vi "Perdite da step carichi.vi"(5 "k0":dbl=1.0 format="%#_13g", 7 "Scorr 0":dbl, 8 "Acqisizioni termica":T4, 9 "Perdite da termica":T6, 10 "Acquisizioni step carichi":T5, 11 "Perdite da prova a vuoto 2":T1) -> (1 "RISULTATI":T2, 2 "Calcoli da step carichi":T3)   [LabVIEW 2019]
uses:
  <vilib>/Analysis/NI_AALPro.lvlib
panel:
  out "Array 4":dbl[](array[numeric])
  out "Array 3":dbl[](array[numeric])
  out "R iniz carico":dbl
  out "slope":dbl
  out "intercept":dbl
  out "XY Graph":cluster{dbl[], "Best Linear Fit":dbl[]}[](graph)
  out "Array 2":dbl[](array[numeric])
  out "Array":dbl[](array[numeric])
  out "size(s) 2":i32
  out "size(s)":i32
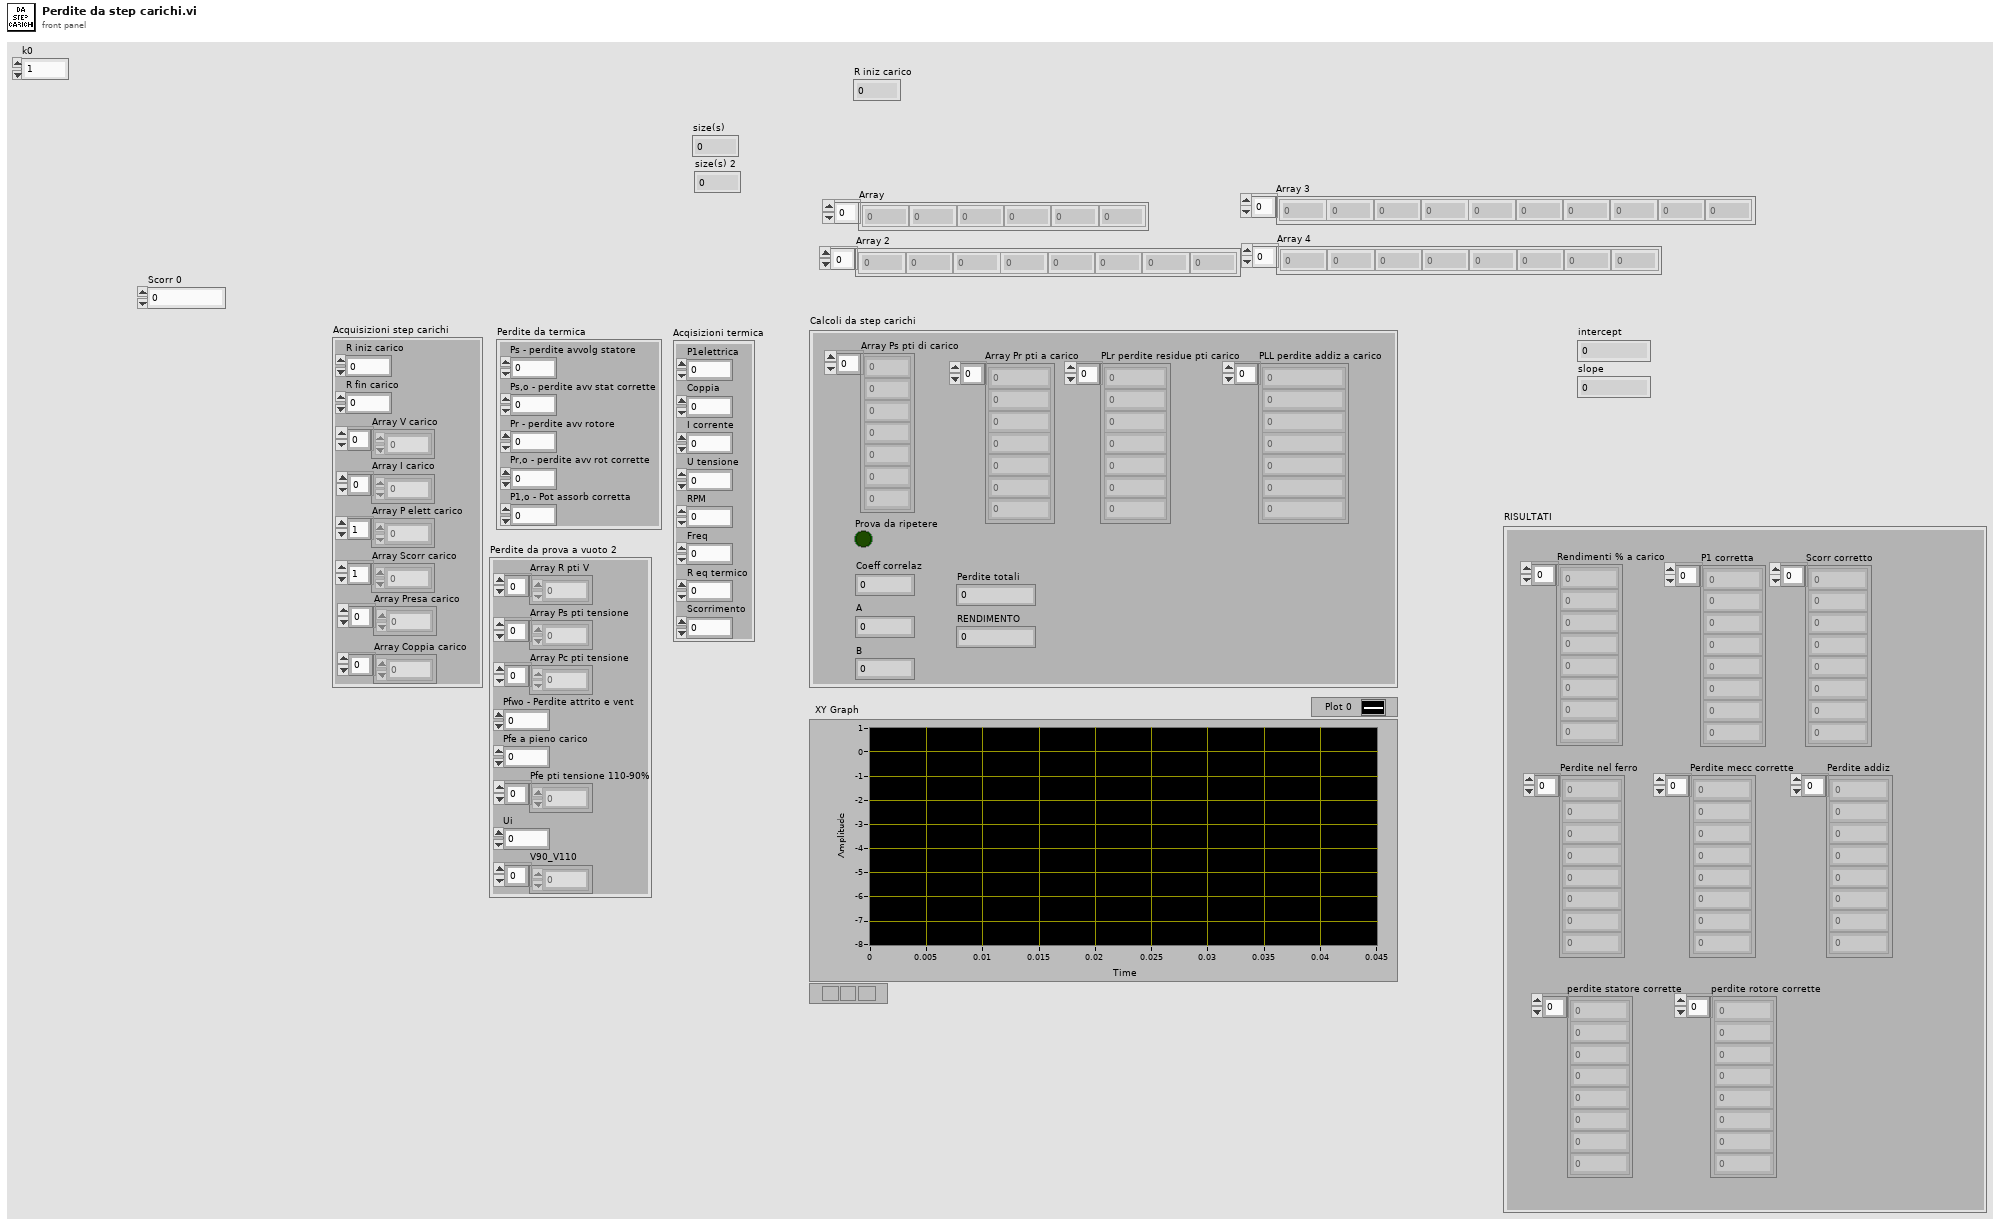
[diagram p1: front panel]
types:
  T1 = cluster{"Array R pti V":dbl[], "Array Ps pti tensione":dbl[], "Array Pc pti tensione":dbl[], "Pfwo - Perdite attrito e vent":dbl, "Pfe a pieno carico":dbl, "Pfe pti tensione 110-90% ":dbl[], "Ui":dbl, "V90_V110":dbl[]}
  T2 = cluster{"Rendimenti % a carico":dbl[], "P1 corretta":dbl[], "Scorr corretto":dbl[], "Perdite nel ferro":dbl[], "Perdite mecc corrette":dbl[], "Perdite addiz":dbl[], "perdite statore corrette":dbl[], "perdite rotore corrette":dbl[]}
  T3 = cluster{"Array Ps pti di carico":dbl[], "Array Pr pti a carico":dbl[], "PLr perdite residue pti carico":dbl[], "A":dbl, "B":dbl, "Coeff correlaz":dbl, "Prova da ripetere":bool, "PLL perdite addiz a carico":dbl[], "Perdite totali":dbl, "RENDIMENTO":dbl}
  T4 = cluster{"P1elettrica":dbl, "Coppia":dbl, "I corrente":dbl, "U tensione":dbl, "RPM":dbl, "Freq":dbl, "R eq termico":dbl, "Scorrimento":dbl}
  T5 = cluster{"R iniz carico":dbl, "R fin carico":dbl, "Array V carico":dbl[], "Array I carico":dbl[], "Array P elett carico":dbl[], "Array Scorr carico":dbl[], "Array Presa carico":dbl[], "Array Coppia carico":dbl[]}
  T6 = cluster{"Ps - perdite avvolg statore":dbl, "Ps,o - perdite avv stat corrette":dbl, "Pr - perdite avv rotore":dbl, "Pr,o - perdite avv rot corrette":dbl, "P1,o - Pot assorb corretta":dbl}
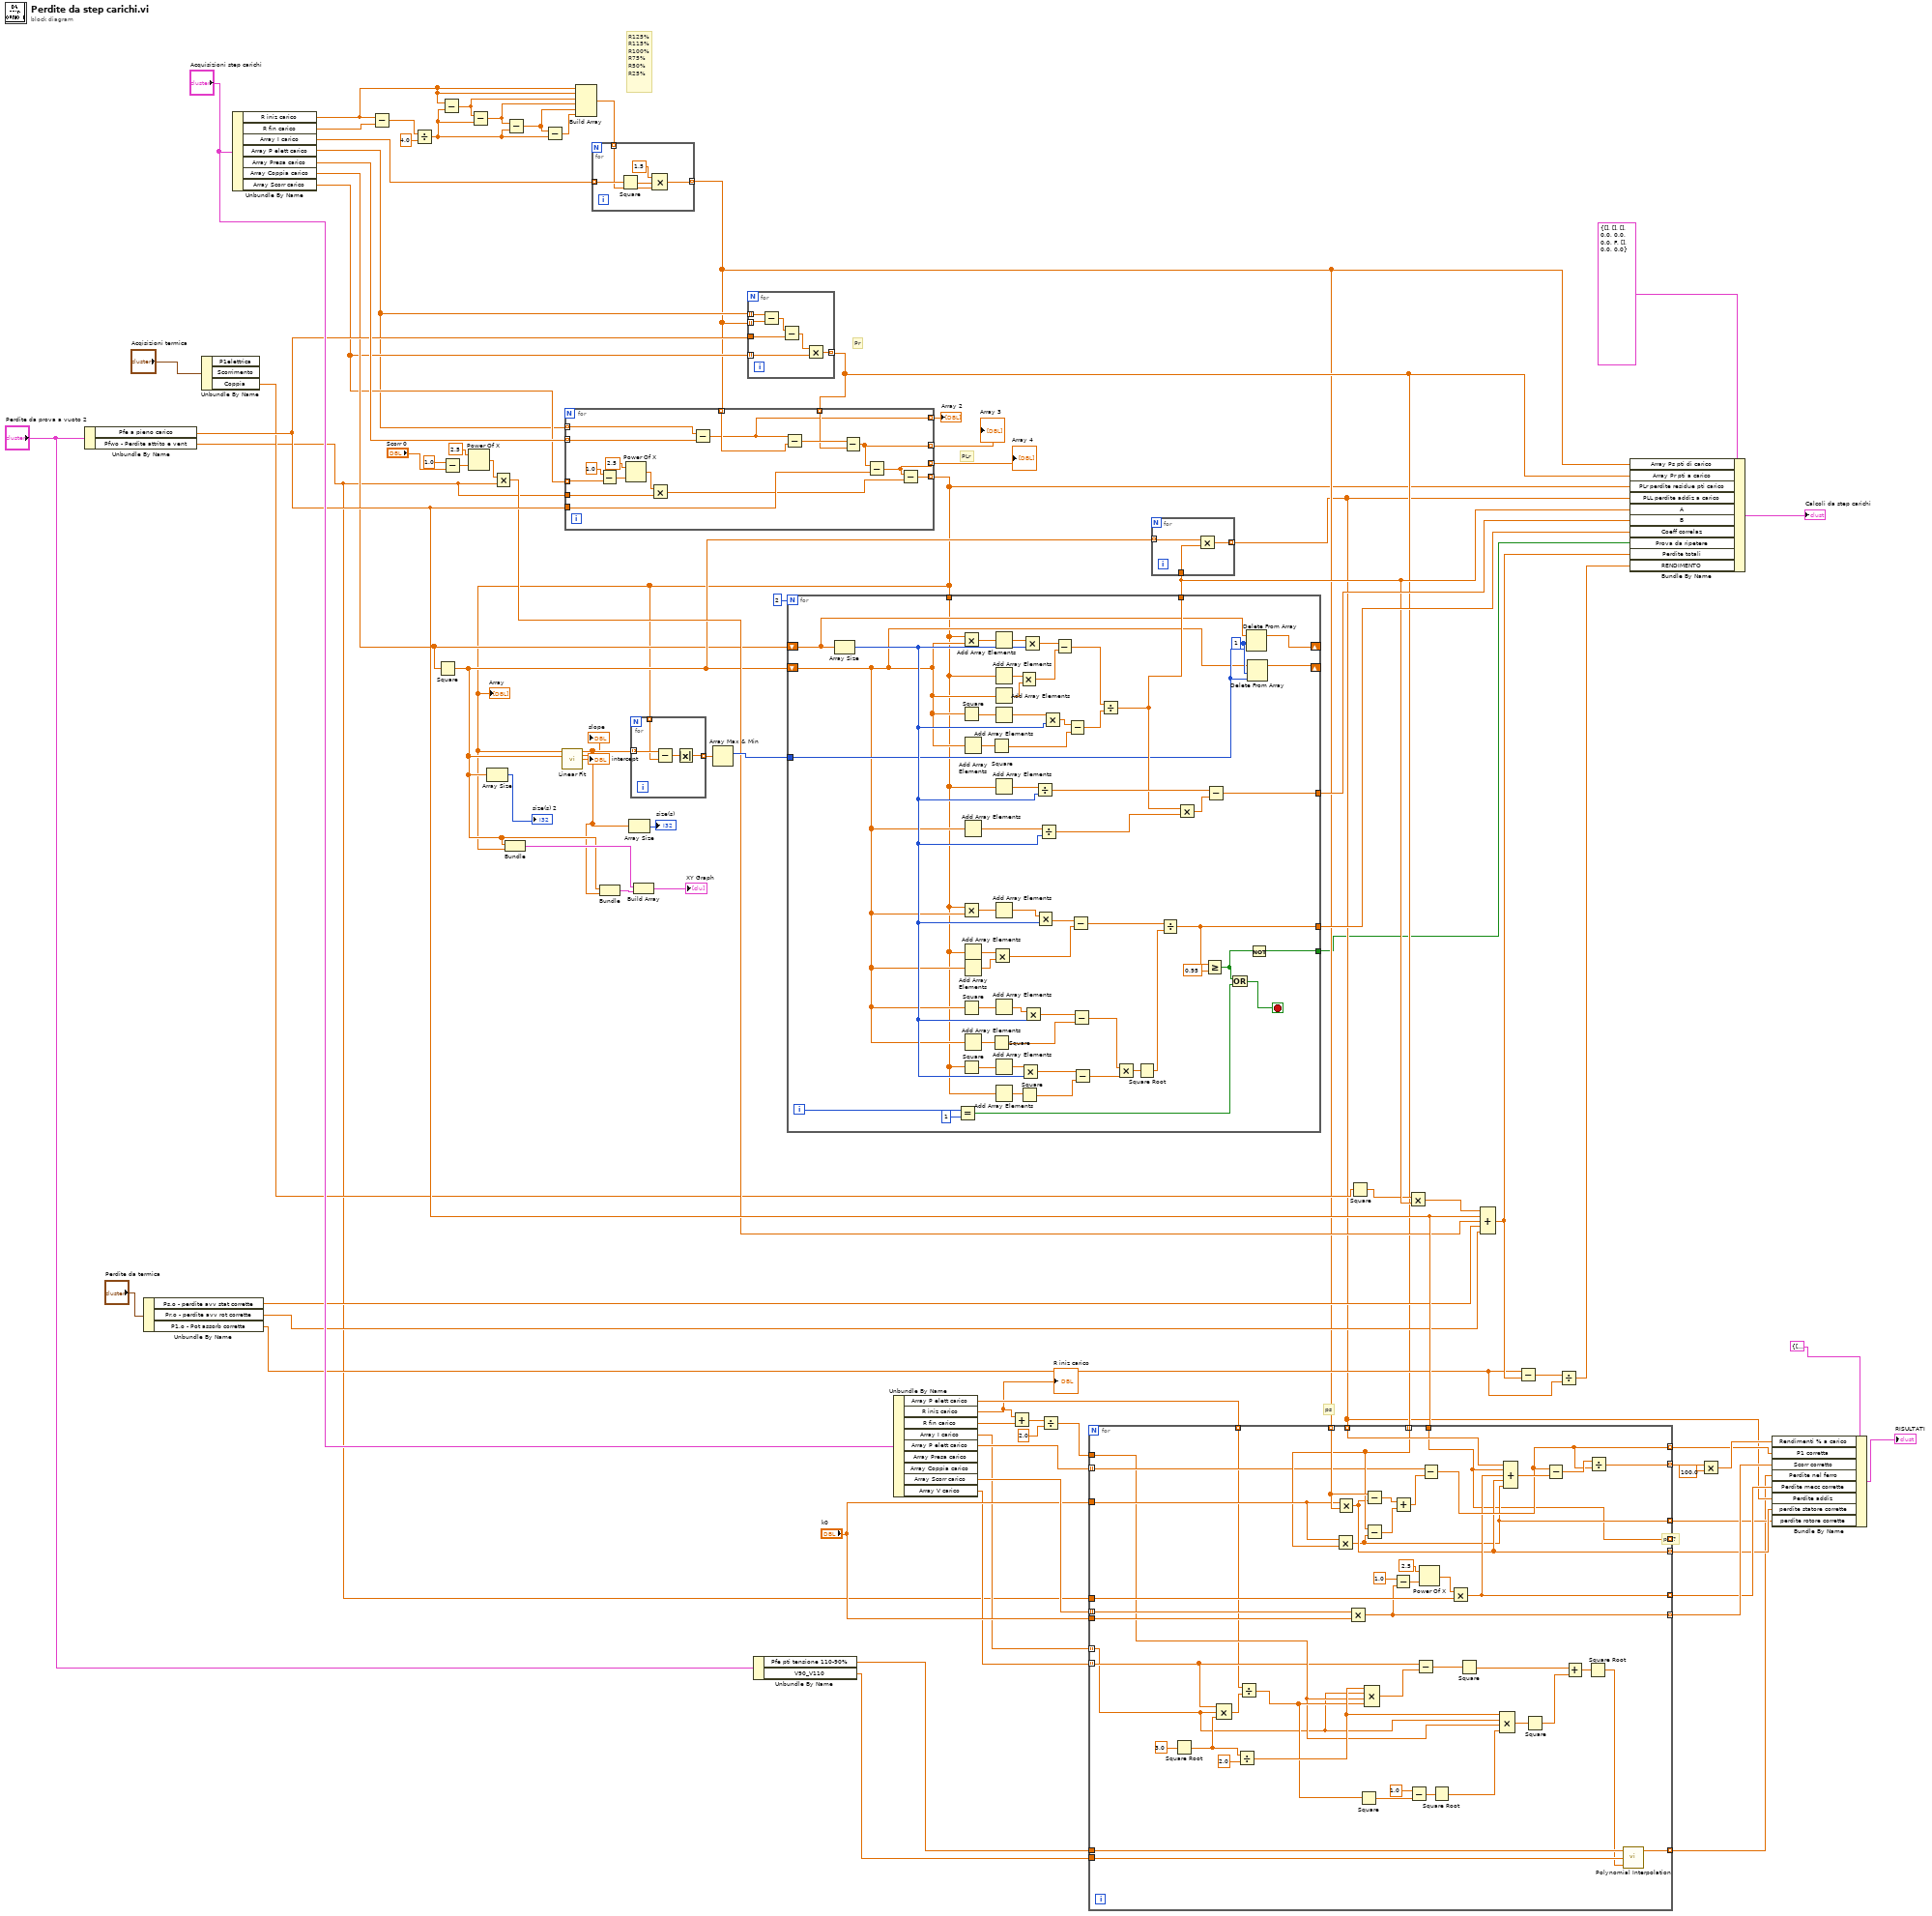
[diagram p0: block diagram]
diagram:
  # "pfe?"
  # "ps"
  # "PLr"
  # "Pr"
  # "R125%\nR115%\nR100%\nR75%\nR50%\nR25%"
  n1 = Unbundle By Name("Perdite da prova a vuoto 2") -> ("Pfe a pieno carico"=w47:dbl, "Pfwo - Perdite attrito e vent"=w1:dbl)
  n2 = Unbundle By Name("Perdite da termica") -> ("Ps,o - perdite avv stat corrette"=w43:dbl, "Pr,o - perdite avv rot corrette"=w42:dbl, "P1,o - Pot assorb corretta"=w41:dbl)
  n3 = Unbundle By Name("Acqisizioni termica") -> ("Coppia"=w45:dbl)  [unwired: 2 out]
  n4 = Unbundle By Name("Acquisizioni step carichi") -> ("R iniz carico"=w70:dbl, "R fin carico"=w69:dbl, "Array I carico"=w68:dbl[], "Array P elett carico"=w34:dbl[], "Array Presa carico"=w65:dbl[], "Array Coppia carico"=w36:dbl[], "Array Scorr carico"=w35:dbl[])
  n5 = Subtract(x=w70, y=w69) -> (x-y=w85:dbl)
  n6 = Divide(x=w85, y=4.0) -> (x/y=w57:dbl)
  n7 = Square(x=w36) -> (x^2=w40:dbl[])
  n8 = Subtract(x=w70, y=w57) -> (x-y=w83:dbl)
  n9 = Subtract(x=1.0, y="Scorr 0") -> (x-y=w79:dbl)
  n10 = Power Of X(1:w79, 2:2.5 ("y")) -> (0:w77:dbl)
  n11 = Subtract(x=w83, y=w57) -> (x-y=w82:dbl)
  n12 = Array Size(array=w40) -> (size(s)=→"size(s) 2":i32)
  n13 = Multiply(x=w77, y=w1) -> (x*y=w46:dbl)
  n14 = Subtract(x=w82, y=w57) -> (x-y=w58:dbl)
  n15 = Subtract(x=w58, y=w57) -> (x-y=w56:dbl)
  n16 = Build Array(w70, w70, w83, w82, w58, w56) -> (w81:dbl[])
  n17 = for {
    tunnel: w68 -> [w89] mode=indexing
    tunnel: w81 -> [w88] mode=indexing
    tunnel: [w87] -> w29 mode=indexing
    n18 = Square(x=w89) -> (x^2=w86:dbl)
    n19 = Compound Arithmetic op=MULTIPLY(1.5 ("value"), w86, w88) -> (w87:dbl)
  }
  n20 = for {
    tunnel: w34 -> [w97] mode=indexing
    tunnel: w29 -> [w96] mode=indexing
    tunnel: w47 -> [w94]
    tunnel: [w91] -> w31 mode=indexing
    tunnel: w35 -> [w92] mode=indexing
    n21 = Subtract(x=w97, y=w96) -> (x-y=w95:dbl)
    n22 = Subtract(x=w95, y=w94) -> (x-y=w93:dbl)
    n23 = Multiply(x=w93, y=w92) -> (x*y=w91:dbl)
  }
  n24 = for {
    tunnel: w34 -> [w114] mode=indexing
    tunnel: w65 -> [w113] mode=indexing
    tunnel: w29 -> [w112] mode=indexing
    tunnel: w31 -> [w110] mode=indexing
    tunnel: w47 -> [w108]
    tunnel: [w109] -> w17 mode=indexing
    tunnel: w35 -> [w103] mode=indexing
    tunnel: w1 -> [w102]
    tunnel: [w100] -> w54 mode=indexing
    tunnel: [w99] -> w3 mode=indexing
    tunnel: [w98] -> w2 mode=indexing
    n25 = Subtract(x=1.0, y=w103) -> (x-y=w105:dbl)
    n26 = Power Of X(1:w105, 2:2.5 ("y")) -> (0:w107:dbl)
    n27 = Multiply(x=w107, y=w102) -> (x*y=w101:dbl)
    n28 = Subtract(x=w114, y=w113) -> (x-y=w100:dbl)
    n29 = Subtract(x=w100, y=w112) -> (x-y=w111:dbl)
    n30 = Subtract(x=w111, y=w110) -> (x-y=w99:dbl)
    n31 = Subtract(x=w99, y=w108) -> (x-y=w98:dbl)
    n32 = Subtract(x=w98, y=w101) -> (x-y=w109:dbl)
  }
  "Array" <- w17
  "Array 2" <- w54
  "Array 3" <- w3
  "Array 4" <- w2
  n33 = Bundle(w40, w17) -> (w53:cluster{dbl[], dbl[]})  [unwired: 1 in]
  n34 = call <vilib>:"Linear Fit.vi"("Y"=w17, "X"=w40) -> ("Best Linear Fit"=w39:dbl[], "slope"=→"slope":dbl, "intercept"=→"intercept":dbl)  [unwired: 9 in, 2 out]
  n35 = Bundle(w40, "Best Linear Fit"=w39) -> (w52:cluster{dbl[], "Best Linear Fit":dbl[]})  [unwired: 1 in]
  n36 = Array Size(array=w39) -> (size(s)=→"size(s)":i32)
  n37 = for {
    tunnel: w39 -> [w118] mode=indexing
    tunnel: w17 -> [w117] mode=indexing
    tunnel: [w115] -> w75 mode=indexing
    n38 = Subtract(x=w118, y=w117) -> (x-y=w116:dbl)
    n39 = Absolute Value(x=w116) -> (abs(x)=w115:dbl)
  }
  n40 = Build Array(w53, w52) -> (→"XY Graph":cluster{dbl[], "Best Linear Fit":dbl[]}[])
  n41 = Array Max & Min(array=w75) -> (max index (indices)=w74:i32)  [unwired: 3 out]
  n42 = Unbundle By Name("Perdite da prova a vuoto 2") -> ("Pfe pti tensione 110-90%"=w12:dbl[], "V90_V110"=w11:dbl[])
  n43 = for {
    N: 2 -> [_]
    tunnel: [w143] -> w48
    tunnel: w17 -> [w123]
    tunnel: [w119] -> w4
    tunnel: [w142] -> w63
    shift-right: [w138] -> _
    shift-left: w36 -> [w139]
    shift-right: [w137] -> _
    shift-left: w40 -> [w131]
    tunnel: w74 -> [w140]
    tunnel: [w128] -> w62
    i -> [w135]
    stop <- w132 stop-if-true
    w141 = 1 ("length")
    n44 = Array Size(array=w139) -> (size(s)=w146:i32)
    n45 = Equal?(x=w135, y=1) -> (x = y?=w133:bool)
    n46 = Square(x=w131) -> (x^2=w130:dbl[])
    n47 = Square(x=w131) -> (x^2=w153:dbl[])
    n48 = Square(x=w123) -> (x^2=w147:dbl[])
    n49 = Multiply(x=w123, y=w131) -> (x*y=w175:dbl[])
    n50 = Multiply(x=w123, y=w131) -> (x*y=w158:dbl[])
    n51 = Add Array Elements(numeric array=w131) -> (sum=w167:dbl)
    n52 = Add Array Elements(numeric array=w131) -> (sum=w162:dbl)
    n53 = Add Array Elements(numeric array=w123) -> (sum=w156:dbl)
    n54 = Add Array Elements(numeric array=w131) -> (sum=w155:dbl)
    n55 = Add Array Elements(numeric array=w131) -> (sum=w150:dbl)
    n56 = Square(x=w167) -> (x^2=w166:dbl)
    n57 = Square(x=w150) -> (x^2=w149:dbl)
    n58 = Multiply(x=w156, y=w155) -> (x*y=w154:dbl)
    n59 = Add Array Elements(numeric array=w175) -> (sum=w174:dbl)
    n60 = Add Array Elements(numeric array=w123) -> (sum=w172:dbl)
    n61 = Add Array Elements(numeric array=w131) -> (sum=w168:dbl)
    n62 = Add Array Elements(numeric array=w130) -> (sum=w129:dbl)
    n63 = Add Array Elements(numeric array=w123) -> (sum=w164:dbl)
    n64 = Add Array Elements(numeric array=w158) -> (sum=w159:dbl)
    n65 = Add Array Elements(numeric array=w153) -> (sum=w152:dbl)
    n66 = Add Array Elements(numeric array=w147) -> (sum=w124:dbl)
    n67 = Add Array Elements(numeric array=w123) -> (sum=w122:dbl)
    n68 = Multiply(x=w172, y=w168) -> (x*y=w171:dbl)
    n69 = Square(x=w122) -> (x^2=w121:dbl)
    n70 = Multiply(x=w124, y=w146) -> (x*y=w145:dbl)
    n71 = Multiply(x=w174, y=w146) -> (x*y=w173:dbl)
    n72 = Multiply(x=w152, y=w146) -> (x*y=w151:dbl)
    n73 = Divide(x=w164, y=w146) -> (x/y=w163:dbl)
    n74 = Multiply(x=w159, y=w146) -> (x*y=w157:dbl)
    n75 = Divide(x=w162, y=w146) -> (x/y=w161:dbl)
    n76 = Multiply(x=w129, y=w146) -> (x*y=w169:dbl)
    n77 = Subtract(x=w173, y=w171) -> (x-y=w170:dbl)
    n78 = Subtract(x=w169, y=w166) -> (x-y=w165:dbl)
    n79 = Subtract(x=w157, y=w154) -> (x-y=w126:dbl)
    n80 = Subtract(x=w151, y=w149) -> (x-y=w148:dbl)
    n81 = Subtract(x=w145, y=w121) -> (x-y=w144:dbl)
    n82 = Divide(x=w170, y=w165) -> (x/y=w143:dbl)
    n83 = Multiply(x=w148, y=w144) -> (x*y=w125:dbl)
    n84 = Square Root(x=w125) -> (sqrt(x)=w127:dbl)
    n85 = Divide(x=w126, y=w127) -> (x/y=w128:dbl)
    n86 = Multiply(x=w143, y=w161) -> (x*y=w160:dbl)
    n87 = Greater Or Equal?(x=w128, y=0.95) -> (x >= y?=w120:bool)
    n88 = Subtract(x=w163, y=w160) -> (x-y=w142:dbl)
    n89 = Or(x=w120, y=w133) -> (x .or. y?=w132:bool)
    n90 = Delete From Array(array=w139, length=w141, index=w140) -> (array with subset deleted=w138:dbl[])  [unwired: 1 out]
    n91 = Delete From Array(array=w131, length=w141, index=w140) -> (array with subset deleted=w137:dbl[])  [unwired: 1 out]
    n92 = Not(x=w120) -> (.not. x?=w119:bool)
  }
  n93 = Unbundle By Name("Acquisizioni step carichi") -> ("Array P elett carico"=w14:dbl[], "R iniz carico"=w9:dbl, "R fin carico"=w6:dbl, "Array I carico"=w15:dbl[], "Array P elett carico"=w33:dbl[], "Array Scorr carico"=w32:dbl[], "Array V carico"=w16:dbl[])  [unwired: 2 out]
  "R iniz carico" <- w9
  n94 = Add(x=w9, y=w6) -> (x+y=w8:dbl)
  n95 = Divide(x=w8, y=2.0) -> (x/y=w5:dbl)
  n96 = for {
    tunnel: w40 -> [w178] mode=indexing
    tunnel: w48 -> [w177]
    tunnel: [w176] -> w20 mode=indexing
    n97 = Multiply(x=w178, y=w177) -> (x*y=w176:dbl)
  }
  n98 = for {
    tunnel: w47 -> [w203]
    tunnel: [w224] -> w26 mode=indexing
    tunnel: w20 -> [w218] mode=indexing
    tunnel: w33 -> [w211] mode=indexing
    tunnel: w1 -> [w219]
    tunnel: w32 -> [w210] mode=indexing
    tunnel: w31 -> [w215] mode=indexing
    tunnel: w29 -> [w217] mode=indexing
    tunnel: "k0" -> [w216]
    tunnel: "k0" -> [w209]
    tunnel: [w208] -> w23 mode=indexing
    tunnel: [w207] -> w22 mode=indexing
    tunnel: [w203] -> _ mode=indexing
    tunnel: [w206] -> w21 mode=indexing
    tunnel: [w205] -> w19 mode=indexing
    tunnel: [w204] -> w18 mode=indexing
    tunnel: w5 -> [w187]
    tunnel: w16 -> [w186] mode=indexing
    tunnel: w15 -> [w184] mode=indexing
    tunnel: w14 -> [w183] mode=indexing
    tunnel: w12 -> [w182]
    tunnel: w11 -> [w181]
    tunnel: [w179] -> w10 mode=indexing
    n99 = Square Root(x=3.0) -> (sqrt(x)=w201:dbl)
    n100 = Compound Arithmetic op=MULTIPLY(w186, w184, w201) -> (w202:dbl)
    n101 = Divide(x=w201, y=2.0) -> (x/y=w196:dbl)
    n102 = Divide(x=w183, y=w202) -> (x/y=w195:dbl)
    n103 = Multiply(x=w216, y=w215) -> (x*y=w204:dbl)
    n104 = Multiply(x=w216, y=w217) -> (x*y=w205:dbl)
    n105 = Multiply(x=w210, y=w209) -> (x*y=w207:dbl)
    n106 = Square(x=w195) -> (x^2=w193:dbl)
    n107 = Subtract(x=w217, y=w205) -> (x-y=w214:dbl)
    n108 = Subtract(x=w215, y=w204) -> (x-y=w213:dbl)
    n109 = Compound Arithmetic op=MULTIPLY(w196, w184, w187, w195) -> (w199:dbl)
    n110 = Subtract(x=1.0, y=w207) -> (x-y=w222:dbl)
    n111 = Add(x=w214, y=w213) -> (x+y=w212:dbl)
    n112 = Subtract(x=1.0, y=w193) -> (x-y=w192:dbl)
    n113 = Subtract(x=w186, y=w199) -> (x-y=w198:dbl)
    n114 = Power Of X(1:w222, 2:2.5 ("y")) -> (0:w220:dbl)
    n115 = Subtract(x=w211, y=w212) -> (x-y=w208:dbl)
    n116 = Square Root(x=w192) -> (sqrt(x)=w191:dbl)
    n117 = Multiply(x=w220, y=w219) -> (x*y=w206:dbl)
    n118 = Square(x=w198) -> (x^2=w197:dbl)
    n119 = Compound Arithmetic op=MULTIPLY(w196, w184, w187, w191) -> (w190:dbl)
    n120 = Compound Arithmetic op=ADD(w218, w203, w206, w205, w204) -> (w225:dbl)
    n121 = Square(x=w190) -> (x^2=w189:dbl)
    n122 = Subtract(x=w208, y=w225) -> (x-y=w226:dbl)
    n123 = Add(x=w197, y=w189) -> (x+y=w188:dbl)
    n124 = Square Root(x=w188) -> (sqrt(x)=w180:dbl)
    n125 = Divide(x=w226, y=w208) -> (x/y=w224:dbl)
    n126 = call <vilib>:"Polynomial Interpolation.vi"("x value"=w180, "X"=w181, "Y"=w182) -> ("interpolation value"=w179:dbl)  [unwired: 2 out]
  }
  n127 = Square(x=w45) -> (x^2=w44:dbl)
  n128 = Multiply(x=w44, y=w48) -> (x*y=w73:dbl)
  n129 = Compound Arithmetic op=ADD(w73, w47, w46, w43, w42) -> (w61:dbl)
  n130 = Subtract(x=w41, y=w61) -> (x-y=w72:dbl)
  n131 = Divide(x=w72, y=w41) -> (x/y=w60:dbl)
  n132 = Bundle By Name(cluster=T3 {"Array Ps pti di carico"=[], "Array Pr pti a carico"=[], "PLr perdite residue pti carico"=[], "A"=0.0, "B"=0.0, "Coeff correlaz"=0.0, "Prova da ripetere"=FALSE, "PLL perdite addiz a carico"=[], "Perdite totali"=0.0, "RENDIMENTO"=0.0} ("Calcoli da step carichi"), "Array Ps pti di carico"=w29, "Array Pr pti a carico"=w31, "PLr perdite residue pti carico"=w17, "PLL perdite addiz a carico"=w20, "A"=w48, "B"=w63, "Coeff correlaz"=w62, "Prova da ripetere"=w4, "Perdite totali"=w61, "RENDIMENTO"=w60) -> (→"Calcoli da step carichi":T3)
  n133 = Multiply(x=w26, y=100.0 ("x")) -> (x*y=w24:dbl[])
  n134 = Bundle By Name(cluster=T2 {"Rendimenti % a carico"=[0.7302451712444388, 0.7575394109341196, 0.7720884225919996, 0.772070279680063, 0.7450543637486186, 0.6500664036979227], "P1 corretta"=[0.7302451712444388, 0.7575394109341196, 0.7720884225919996, 0.772070279680063, 0.7450543637486186, 0.6500664036979227], "Scorr corretto"=[0.7302451712444388, 0.7575394109341196, 0.7720884225919996, 0.772070279680063, 0.7450543637486186, 0.6500664036979227], "Perdite nel ferro"=[0.7302451712444388, 0.7575394109341196, 0.7720884225919996, 0.772070279680063, 0.7450543637486186, 0.6500664036979227], "Perdite mecc corrette"=[0.7302451712444388, 0.7575394109341196, 0.7720884225919996, 0.772070279680063, 0.7450543637486186, 0.6500664036979227], "Perdite addiz"=[0.7302451712444388, 0.7575394109341196, 0.7720884225919996, 0.772070279680063, 0.7450543637486186, 0.6500664036979227], "perdite statore corrette"=[0.7302451712444388, 0.7575394109341196, 0.7720884225919996, 0.772070279680063, 0.7450543637486186, 0.6500664036979227], "perdite rotore corrette"=[0.7302451712444388, 0.7575394109341196, 0.7720884225919996, 0.772070279680063, 0.7450543637486186, 0.6500664036979227]} ("RISULTATI"), "Rendimenti % a carico"=w24, "P1 corretta"=w23, "Scorr corretto"=w22, "Perdite nel ferro"=w10, "Perdite mecc corrette"=w21, "Perdite addiz"=w20, "perdite statore corrette"=w19, "perdite rotore corrette"=w18) -> (→"RISULTATI":T2)
